vi "Modbus_subvi.vi"(11 "Modbus master in":refnum<class "Modbus Master.lvclass">) -> (0 "Output 2 temp alarm":string, 1 "Output 3 temp alarm":string, 2 "Controller output 3 alarm":string, 3 "Controller output 2 alarm":string, 4 "Output 1 temp alarm":string, 5 "Controller output 1 alarm":string, 6 "Variables voltage":string, 8 "Modbus master out":refnum<class "Modbus Master.lvclass">)   [LabVIEW 2017]
uses:
  <vilib>/NI/Modbus Library/API/Master/Modbus Master.lvclass
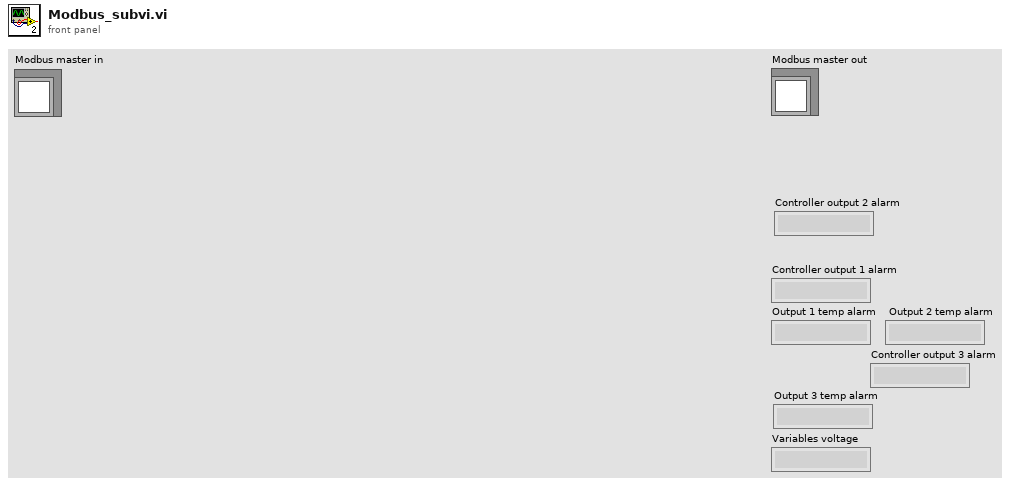
[diagram p1: front panel]
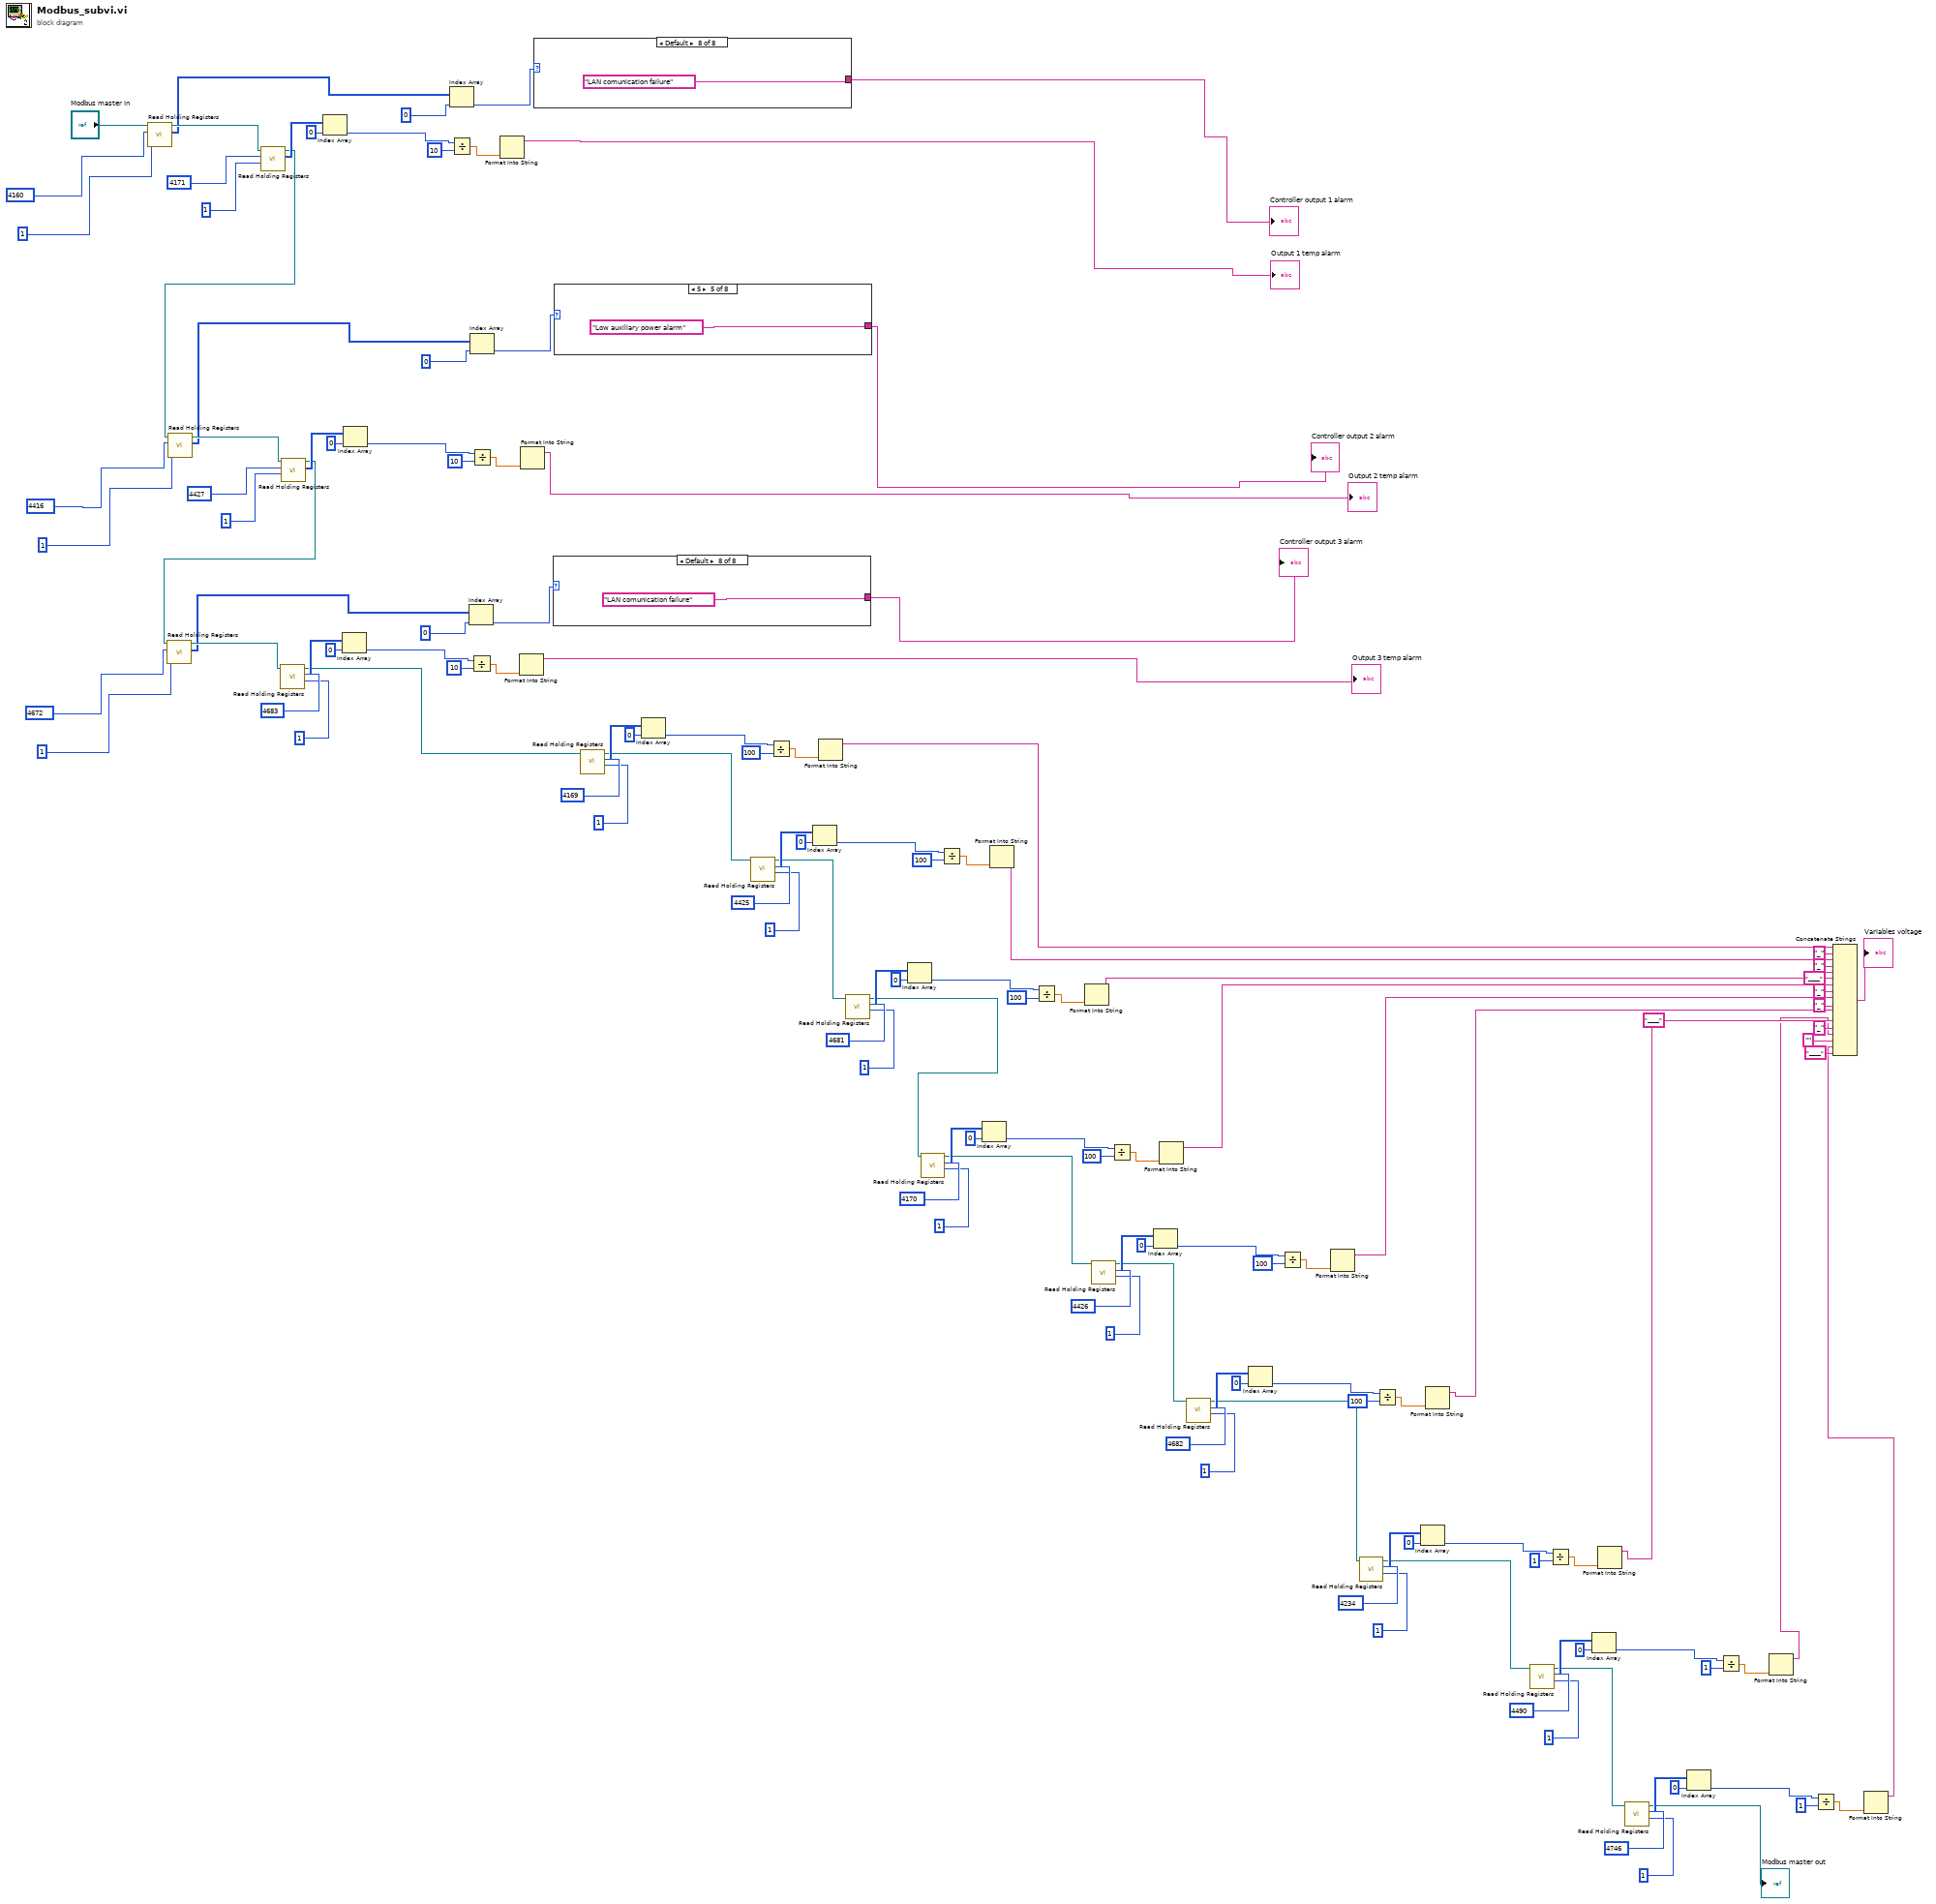
[diagram p0: block diagram]
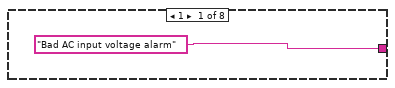
[diagram p2: hidden frame]
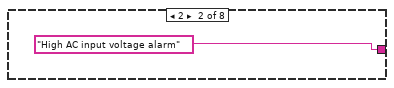
[diagram p3: hidden frame]
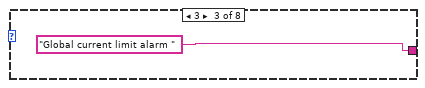
[diagram p4: hidden frame]
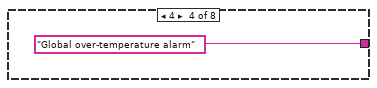
[diagram p5: hidden frame]
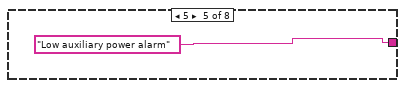
[diagram p6: hidden frame]
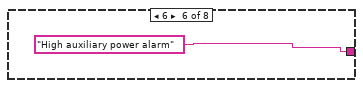
[diagram p7: hidden frame]
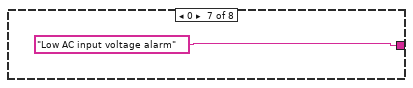
[diagram p8: hidden frame]
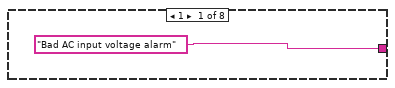
[diagram p9: hidden frame]
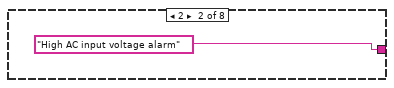
[diagram p10: hidden frame]
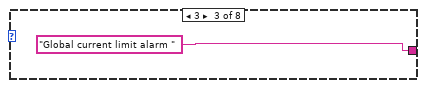
[diagram p11: hidden frame]
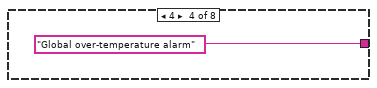
[diagram p12: hidden frame]
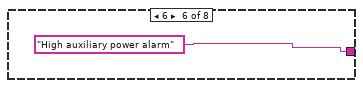
[diagram p13: hidden frame]
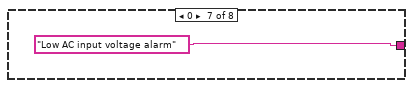
[diagram p14: hidden frame]
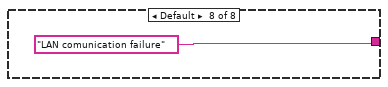
[diagram p15: hidden frame]
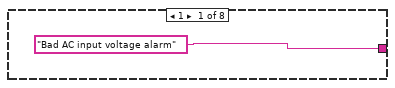
[diagram p16: hidden frame]
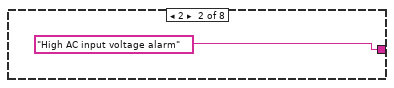
[diagram p17: hidden frame]
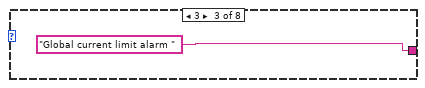
[diagram p18: hidden frame]
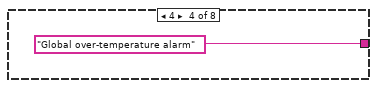
[diagram p19: hidden frame]
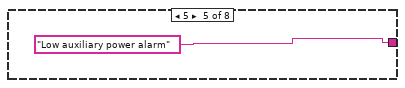
[diagram p20: hidden frame]
diagram:
  n1 = call-dynamic "Read Holding Registers.vi"("number of inputs"=u16 1, "starting address"=u32 4160, "Modbus master in"="Modbus master in") -> ("register values"=w135:u16[], "Modbus master out"=w138:refnum<class "Modbus Master.lvclass">)  [unwired: 6 in, 1 out]
  n2 = call-dynamic "Read Holding Registers.vi"("number of inputs"=u16 1, "starting address"=u32 4171, "Modbus master in"=w138) -> ("register values"=w132:u16[], "Modbus master out"=w114:refnum<class "Modbus Master.lvclass">)  [unwired: 6 in, 1 out]
  n3 = call-dynamic "Read Holding Registers.vi"("number of inputs"=u16 1, "starting address"=u32 4416, "Modbus master in"=w114) -> ("register values"=w122:u16[], "Modbus master out"=w125:refnum<class "Modbus Master.lvclass">)  [unwired: 6 in, 1 out]
  n4 = call-dynamic "Read Holding Registers.vi"("number of inputs"=u16 1, "starting address"=u32 4427, "Modbus master in"=w125) -> ("register values"=w119:u16[], "Modbus master out"=w100:refnum<class "Modbus Master.lvclass">)  [unwired: 6 in, 1 out]
  n5 = call-dynamic "Read Holding Registers.vi"("number of inputs"=u16 1, "starting address"=u32 4672, "Modbus master in"=w100) -> ("register values"=w108:u16[], "Modbus master out"=w111:refnum<class "Modbus Master.lvclass">)  [unwired: 6 in, 1 out]
  n6 = call-dynamic "Read Holding Registers.vi"("number of inputs"=u16 1, "starting address"=u32 4683, "Modbus master in"=w111) -> ("register values"=w105:u16[], "Modbus master out"=w71:refnum<class "Modbus Master.lvclass">)  [unwired: 6 in, 1 out]
  n7 = Index Array(array=w132, index=0) -> (element=w130:u16)
  n8 = Index Array(array=w105, index=0) -> (element=w103:u16)
  n9 = Index Array(array=w119, index=0) -> (element=w117:u16)
  n10 = Index Array(array=w135, index=0) -> (element=w133:u16)
  n11 = Divide(x=w130, y=u16 10) -> (x/y=w128:dbl)
  n12 = Index Array(array=w108, index=0) -> (element=w106:u16)
  n13 = Index Array(array=w122, index=0) -> (element=w120:u16)
  n14 = Divide(x=w103, y=u16 10) -> (x/y=w101:dbl)
  n15 = Divide(x=w117, y=u16 10) -> (x/y=w115:dbl)
  n16 = Format Into String(w128) -> (resulting string=→"Output 1 temp alarm":string)  [unwired: 3 in, 1 out]
  n17 = Format Into String(w101) -> (resulting string=→"Output 3 temp alarm":string)  [unwired: 3 in, 1 out]
  n18 = Format Into String(w115) -> (resulting string=→"Output 2 temp alarm":string)  [unwired: 3 in, 1 out]
  n19 = case shown="Default" w133 {
    tunnel: ["Bad AC input voltage alarm" "High AC input voltage alarm" "Global current limit alarm " "Global over-temperature alarm" "Low auxiliary power alarm" "High auxiliary power alarm" "Low AC input voltage alarm" "LAN comunication failure"] -> w99
    frame 1 {
    }
    frame 2 {
    }
    frame 3 {
    }
    frame 4 {
    }
    frame 5 {
    }
    frame 6 {
    }
    frame 0 {
    }
    frame Default {
    }
  }
  "Controller output 1 alarm" <- w99
  n20 = case shown="Default" w106 {
    tunnel: ["Bad AC input voltage alarm" "High AC input voltage alarm" "Global current limit alarm " "Global over-temperature alarm" "Low auxiliary power alarm" "High auxiliary power alarm" "Low AC input voltage alarm" "LAN comunication failure"] -> w95
    frame 1 {
    }
    frame 2 {
    }
    frame 3 {
    }
    frame 4 {
    }
    frame 5 {
    }
    frame 6 {
    }
    frame 0 {
    }
    frame Default {
    }
  }
  "Controller output 3 alarm" <- w95
  n21 = case shown="5" w120 {
    tunnel: ["Bad AC input voltage alarm" "High AC input voltage alarm" "Global current limit alarm " "Global over-temperature alarm" "Low auxiliary power alarm" "High auxiliary power alarm" "Low AC input voltage alarm" "LAN comunication failure"] -> w97
    frame 1 {
    }
    frame 2 {
    }
    frame 3 {
    }
    frame 4 {
    }
    frame 5 {
    }
    frame 6 {
    }
    frame 0 {
    }
    frame Default {
    }
  }
  "Controller output 2 alarm" <- w97
  n22 = call-dynamic "Read Holding Registers.vi"("number of inputs"=u16 1, "starting address"=u32 4169, "Modbus master in"=w71) -> ("register values"=w90:u16[], "Modbus master out"=w70:refnum<class "Modbus Master.lvclass">)  [unwired: 6 in, 1 out]
  n23 = Index Array(array=w90, index=0) -> (element=w88:u16)
  n24 = call-dynamic "Read Holding Registers.vi"("number of inputs"=u16 1, "starting address"=u32 4425, "Modbus master in"=w70) -> ("register values"=w83:u16[], "Modbus master out"=w69:refnum<class "Modbus Master.lvclass">)  [unwired: 6 in, 1 out]
  n25 = Divide(x=w88, y=u16 100) -> (x/y=w86:dbl)
  n26 = Index Array(array=w83, index=0) -> (element=w81:u16)
  n27 = Format Into String(w86) -> (resulting string=w68:string)  [unwired: 3 in, 1 out]
  n28 = call-dynamic "Read Holding Registers.vi"("number of inputs"=u16 1, "starting address"=u32 4681, "Modbus master in"=w69) -> ("register values"=w76:u16[], "Modbus master out"=w39:refnum<class "Modbus Master.lvclass">)  [unwired: 6 in, 1 out]
  n29 = Index Array(array=w76, index=0) -> (element=w74:u16)
  n30 = call-dynamic "Read Holding Registers.vi"("number of inputs"=u16 1, "starting address"=u32 4170, "Modbus master in"=w39) -> ("register values"=w60:u16[], "Modbus master out"=w41:refnum<class "Modbus Master.lvclass">)  [unwired: 6 in, 1 out]
  n31 = Divide(x=w81, y=u16 100) -> (x/y=w79:dbl)
  n32 = Index Array(array=w60, index=0) -> (element=w58:u16)
  n33 = Format Into String(w79) -> (resulting string=w65:string)  [unwired: 3 in, 1 out]
  n34 = Divide(x=w74, y=u16 100) -> (x/y=w72:dbl)
  n35 = Format Into String(w72) -> (resulting string=w66:string)  [unwired: 3 in, 1 out]
  n36 = call-dynamic "Read Holding Registers.vi"("number of inputs"=u16 1, "starting address"=u32 4426, "Modbus master in"=w41) -> ("register values"=w53:u16[], "Modbus master out"=w40:refnum<class "Modbus Master.lvclass">)  [unwired: 6 in, 1 out]
  n37 = Divide(x=w58, y=u16 100) -> (x/y=w56:dbl)
  n38 = Index Array(array=w53, index=0) -> (element=w51:u16)
  n39 = Format Into String(w56) -> (resulting string=w12:string)  [unwired: 3 in, 1 out]
  n40 = call-dynamic "Read Holding Registers.vi"("number of inputs"=u16 1, "starting address"=u32 4682, "Modbus master in"=w40) -> ("register values"=w46:u16[], "Modbus master out"=w15:refnum<class "Modbus Master.lvclass">)  [unwired: 6 in, 1 out]
  n41 = Index Array(array=w46, index=0) -> (element=w44:u16)
  n42 = Divide(x=w51, y=u16 100) -> (x/y=w49:dbl)
  n43 = Format Into String(w49) -> (resulting string=w11:string)  [unwired: 3 in, 1 out]
  n44 = call-dynamic "Read Holding Registers.vi"("number of inputs"=u16 1, "starting address"=u32 4234, "Modbus master in"=w15) -> ("register values"=w36:u16[], "Modbus master out"=w17:refnum<class "Modbus Master.lvclass">)  [unwired: 6 in, 1 out]
  n45 = Divide(x=w44, y=u16 100) -> (x/y=w42:dbl)
  n46 = Index Array(array=w36, index=0) -> (element=w34:u16)
  n47 = Format Into String(w42) -> (resulting string=w10:string)  [unwired: 3 in, 1 out]
  n48 = call-dynamic "Read Holding Registers.vi"("number of inputs"=u16 1, "starting address"=u32 4490, "Modbus master in"=w17) -> ("register values"=w29:u16[], "Modbus master out"=w16:refnum<class "Modbus Master.lvclass">)  [unwired: 6 in, 1 out]
  n49 = Divide(x=w34, y=u16 1) -> (x/y=w32:dbl)
  n50 = Index Array(array=w29, index=0) -> (element=w27:u16)
  n51 = Format Into String(w32) -> (resulting string=w6:string)  [unwired: 3 in, 1 out]
  n52 = call-dynamic "Read Holding Registers.vi"("number of inputs"=u16 1, "starting address"=u32 4746, "Modbus master in"=w16) -> ("register values"=w22:u16[], "Modbus master out"=→"Modbus master out":refnum<class "Modbus Master.lvclass">)  [unwired: 6 in, 1 out]
  n53 = Index Array(array=w22, index=0) -> (element=w20:u16)
  n54 = Divide(x=w27, y=u16 1) -> (x/y=w25:dbl)
  n55 = Format Into String(w25) -> (resulting string=w2:string)  [unwired: 3 in, 1 out]
  n56 = Divide(x=w20, y=u16 1) -> (x/y=w18:dbl)
  n57 = Format Into String(w18) -> (resulting string=w1:string)  [unwired: 3 in, 1 out]
  n58 = Concatenate Strings(w68, "_" ("string"), w65, "_" ("string"), w66, "____" ("string"), w12, "_" ("string"), w11, "_" ("string"), w10, "____" ("string"), w6, "_" ("string"), w2, "" ("string"), w1, "____" ("string")) -> (→"Variables voltage":string)
